vi "Is Dispense Boolean.vi"(8 "error in (no error)":errorcluster, 11 "Routine in":refnum<class "Routine.lvclass">) -> (0 "error out":errorcluster, 2 "Is Dispense?":bool, 3 "Routine out":refnum<class "Routine.lvclass">)   [LabVIEW 2019, in "Routine.lvclass"]
uses:
  Routine.lvclass
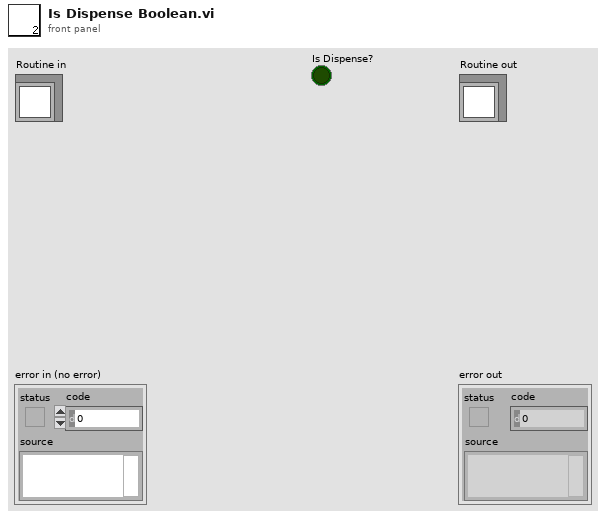
[diagram p1: front panel]
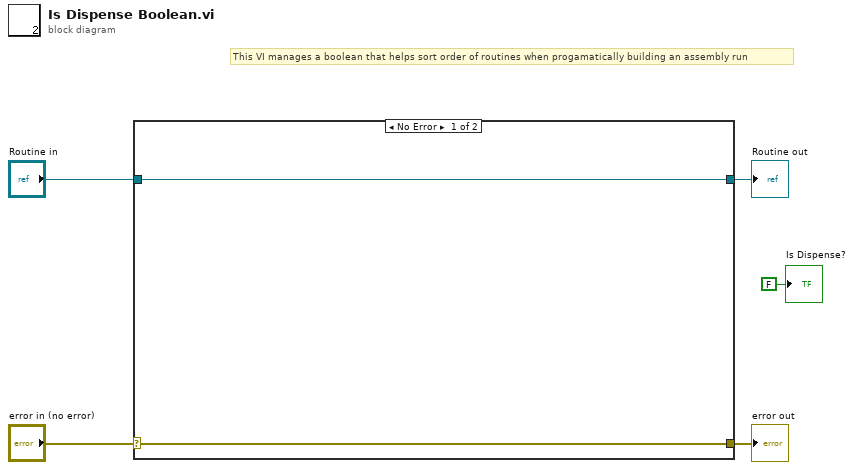
[diagram p0: block diagram]
diagram:
  # "This VI manages a boolean that helps sort order of routines when progamatically building an assembly run"
  n1 = case shown="No Error" "error in (no error)" {
    selector: "error in (no error)" -> [w6 w9]
    tunnel: [w6 w9] -> w4
    tunnel: [w7 w8] -> w2
    tunnel: "Routine in" -> [w7 w8]
    frame No Error {
    }
    frame Error {
    }
  }
  "error out" <- w4
  "Routine out" <- w2
  "Is Dispense?" <- FALSE
